vi "Lab Maximos y Minimos.vi"() -> ()   [LabVIEW 2018]
uses:
  <vilib>/Analysis/baseanly.llb/Mean (DBL).vi
  <vilib>/Analysis/NI_AALBase.lvlib
panel:
  in  "x":bool
  out "mean":dbl format="%0.2f"
  out "Minimo Indexado":i32
  out "Maximo Indexado":i32
  out "Minimo":dbl
  out "Maximo":dbl
  out "Array":dbl[](array[numeric])
  in  "Knob":dbl(knob) scale=0.0..10.0
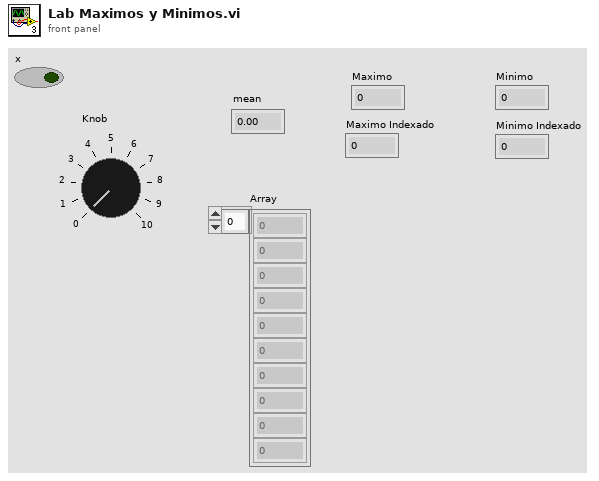
[diagram p1: front panel]
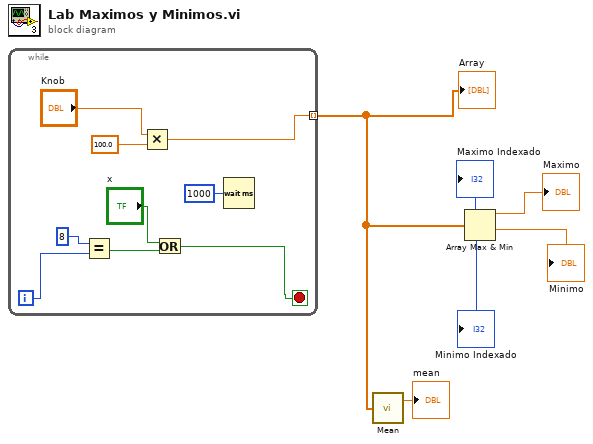
[diagram p0: block diagram]
diagram:
  n1 = while {
    tunnel: [w13] -> w1 mode=indexing
    i -> [w12]
    stop <- w10 stop-if-true
    n2 = Equal?(x=8, y=w12) -> (x = y?=w9:bool)
    n3 = Multiply(x="Knob", y=100.0) -> (x*y=w13:dbl)
    n4 = Or(x="x", y=w9) -> (x .or. y?=w10:bool)
    n5 = Wait (ms)(milliseconds to wait=u32 1000) -> ()  [unwired: 1 out]
  }
  "Array" <- w1
  n6 = call-poly <vilib>:"Mean.vi"("X"=w1) -> ("mean"=→"mean":dbl)  [unwired: 1 out]
  n7 = Array Max & Min(array=w1) -> (max value=→"Maximo":dbl, max index (indices)=→"Maximo Indexado":i32, min value=→"Minimo":dbl, min index (indices)=→"Minimo Indexado":i32)
